vi "Sine Plug In.vi"(9 "Parameters":variant, 10 "Frequency":dbl, 11 "Amplitude":dbl) -> (3 "Signal out":waveform(dbl))   [LabVIEW 2009]
doc: "This is a plug in that is called by the main VI in the exercise.\n\nAAL 9/09"
uses:
  <vilib>/measure/NI_MABase.lvlib
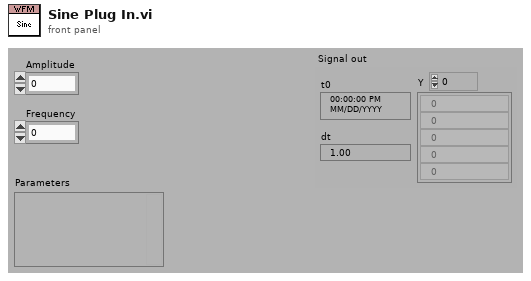
[diagram p1: front panel]
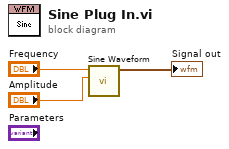
[diagram p0: block diagram]
diagram:
  n1 = call <vilib>:"Sine Waveform.vi"("amplitude"="Amplitude", "frequency"="Frequency") -> ("signal out"=→"Signal out":waveform(dbl))  [unwired: 5 in, 4 out]
